vi "命令字变换.vi"(2 "error in (no error)":errorcluster caption="错误输入（无错误）", 3 "命令字参数":dbl=42.0, 4 "命令字":string(combo)) -> (0 "error out":errorcluster caption="错误输出", 1 "Hex指令":u32[](array[numeric]) format="%.0x")   [LabVIEW 2015, in "MSP6715.lvlib"]
uses:
  MSP6715.lvlib
panel:
  # "(28H/29H)设置或读取负载模式\n负载模式（0为CC, 1为输出CV, 2为CW, 3为CR）"
  # "(2AH/2BH)设置或读取负载的定电流值\n(2CH/2DH)设置或读取负载的定电压值\n(2EH/2FH)设置或读取负载的定功率值\n(30H/31H)设置或读取负载的定电阻值"
  # "(5DH/5EH)设置或读取负载的工作模式\n工作模式(0为FIXED,1为SHORT,2为TRANSITION,3为\nLIST,4为BATTERY)"
  # "(5FH)读取负载的输入电压, 输入电流, 输入功率及相关状态"
  # "(56H/57H)设置或读取负载的远程测量模式的状态"
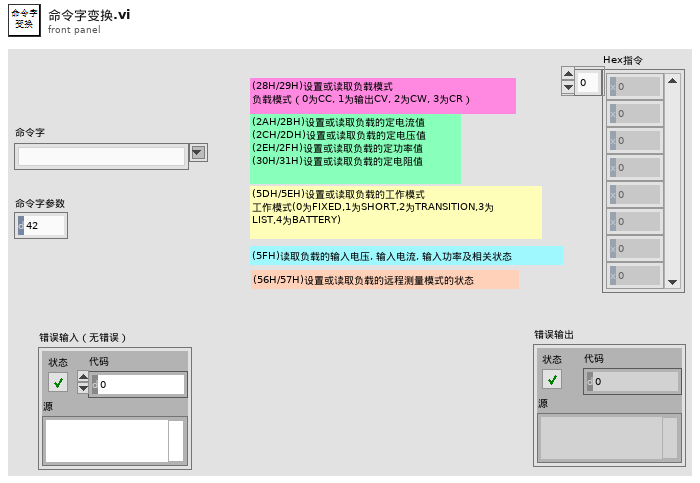
[diagram p1: front panel]
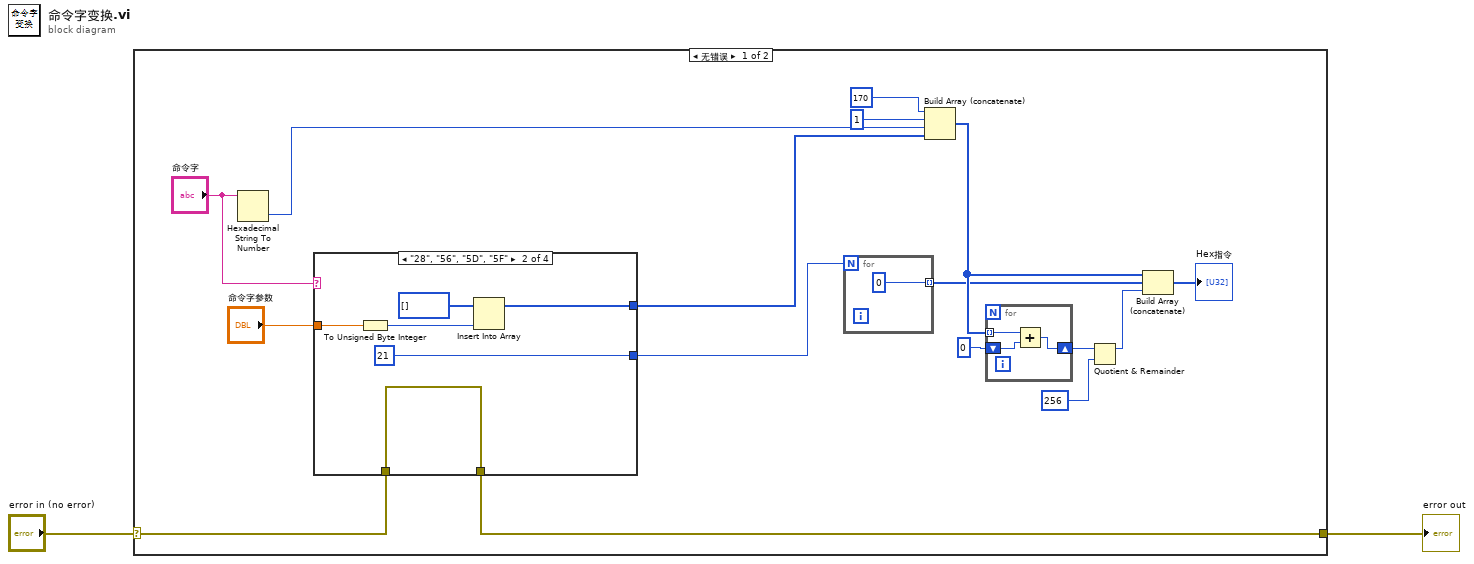
[diagram p0: block diagram]
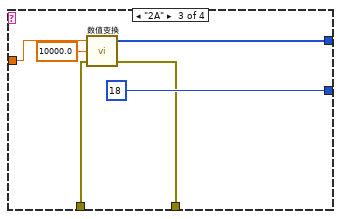
[diagram p3: hidden frame]
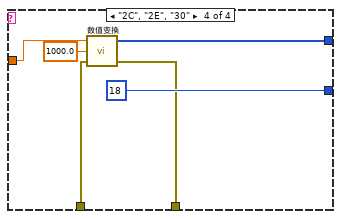
[diagram p4: hidden frame]
diagram:
  n1 = case shown="无错误" "error in (no error)" {
    selector: "error in (no error)" -> [w5 w42]
    tunnel: [w4 w42] -> w1
    frame No Error {
      n2 = Hexadecimal String To Number(string="命令字") -> (number=w10:u32)  [unwired: 2 in, 1 out]
      n3 = case shown="\"28\", \"56\", \"5D\", \"5F\"" "命令字" {
        tunnel: [_ w22 w29 w35] -> w8
        tunnel: [_ 21 18 18] -> w7
        tunnel: "命令字参数" -> [_ w24 w30 w36]
        tunnel: w5 -> [w19 w20 w28 w34]
        tunnel: [w19 w20 w27 w33] -> w4
        frame "0", Default {
        }
        frame "28", "56", "5D", "5F" {
          n4 = To Unsigned Byte Integer(number=w24) -> (unsigned 8bit integer=w23:u8)
          n5 = Insert Into Array(array=u8[] [], new element=w23) -> (w22:u8[])  [unwired: 1 in]
        }
        frame "2A" {
          n6 = call "数值变换.vi"("error in (no error)"=w28, "比例"=10000.0, "数值"=w30) -> ("error out"=w27:errorcluster, "数值变换输出"=w29:u32[])  [unwired: 1 in]
        }
        frame "2C", "2E", "30" {
          n7 = call "数值变换.vi"("error in (no error)"=w34, "比例"=1000.0, "数值"=w36) -> ("error out"=w33:errorcluster, "数值变换输出"=w35:u32[])  [unwired: 1 in]
        }
      }
      n8 = for {
        N: w7 -> [_]
        tunnel: [0] -> w13 mode=indexing
      }
      n9 = Build Array (concatenate)(170, 1, w10, w8) -> (w14:u32[])
      n10 = for {
        tunnel: w14 -> [w40] mode=indexing
        shift-right: [w38] -> w16
        shift-left: u32 0 ("y") -> [w39]
        n11 = Add(x=w40, y=w39) -> (x+y=w38:u32)
      }
      n12 = Quotient & Remainder(x=w16, y=u32 256) -> (x-y*floor(x/y)=w12:u32)  [unwired: 1 out]
      n13 = Build Array (concatenate)(w14, w13, w12) -> (→"Hex指令":u32[])
    }
    frame Error {
    }
  }
  "error out" <- w1
